vi "PicoScope4000aIsReady.vi"(8 "error in (no error)":errorcluster, 11 "handle in":i16) -> (0 "error out":errorcluster, 3 "handle out":i16, 6 "ready":i16)   [LabVIEW 2009]
doc: "Calls sIsReady"
uses:
  ps4000a.dll
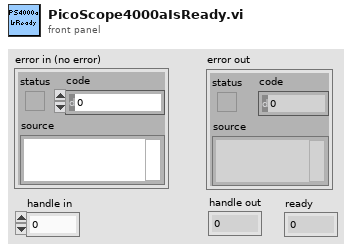
[diagram p1: front panel]
types:
  T1 = cluster{"status":bool, "code":u32, "source":string}
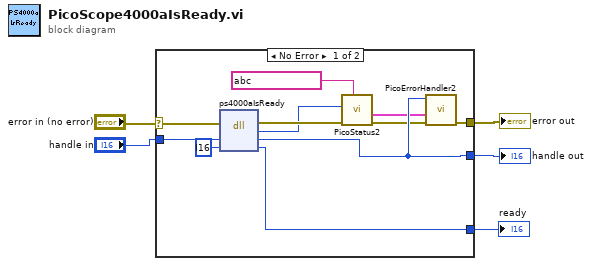
[diagram p0: block diagram]
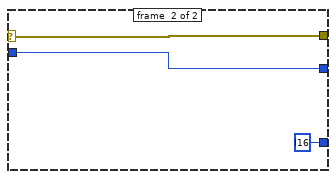
[diagram p2: hidden frame]
diagram:
  n1 = case shown="No Error" "error in (no error)" {
    selector: "error in (no error)" -> [w15 w18]
    tunnel: "handle in" -> [w16 w19]
    tunnel: [w14 w19] -> w5
    tunnel: [w9 w18] -> w4
    tunnel: [w12 i16 ? ("ready")] -> w3
    frame #0 {
      n2 = dll-call lib="ps4000a.dll" fn="ps4000aIsReady" ("ps3000.dll:_ps3000_open_unit@0")(error in=w15, "handle"=w16, "ready"=i16 ?) -> (error out=w11:errorcluster, "PICO_STATUS"=w6:u32, "handle"=w14:i16, "ready"=w12:i16)  [unwired: 2 in, 1 out]
      n3 = call "PicoStatus2.vi"("PICO source"=string ? ("source"), "Error in"=w11, "PICO STATUS"=w6) -> ("error out"=w10:errorcluster, "PICO_STATUS out"=w8:T1)  [unwired: 5 in]
      n4 = call "PicoErrorHandler2.vi"("error in (no error)"=w10, "PICO_STATUS in"=w8, "handle In"=w14) -> ("error out"=w9:errorcluster)  [unwired: 8 in]
    }
    frame #1 {
    }
  }
  "error out" <- w4
  "handle out" <- w5
  "ready" <- w3
